vi "Six Lead ECG Monitor.vi"() -> ()   [LabVIEW 2013]
uses:
  SerialReadStateEnum.ctl
  <vilib>/Utility/file.llb/Write To Spreadsheet File (DBL).vi
  <vilib>/Instr/_visa.llb/VISA Configure Serial Port (Instr).vi
panel:
  out "unsigned byte array":u8[](array[numeric])
  out "size(s)":i32[](array[numeric])
  out "Saved File Path":path
  in  "File Name":string="ecgEarlobe2.txt"
  out "Sync 0":u8=165
  out "Sync 1":u8=90
  out "Protocol Version":u8=2
  out "End Packet":u8=1
  out "Parity":u16(ring) items=["None", "Odd", "Even", "Mark", "Space"]
  out "Stop Bits":u16(ring)=10 items=["1.0"=10, "1.5"=15, "2.0"=20]
  out "Flow Control":u16(ring) items=["None"=0, "XON/XOFF"=1, "RTS/CTS"=2, "DTR/DSR"=4]
  out "Current State":T1
  out "ECG/\nEMG":cluster{u16, u16, u16, u16, u16, u16}(graph)
  out "Count":u8
  out "Byte Count":u32=17
  in  "Stop":bool
  out "Data Bits":u16=8 min=5 max=8 step=1
  in  "VISA resource name":refnum<visa-resource-name>="COM3"
  out "Baud Rate":u32=57600
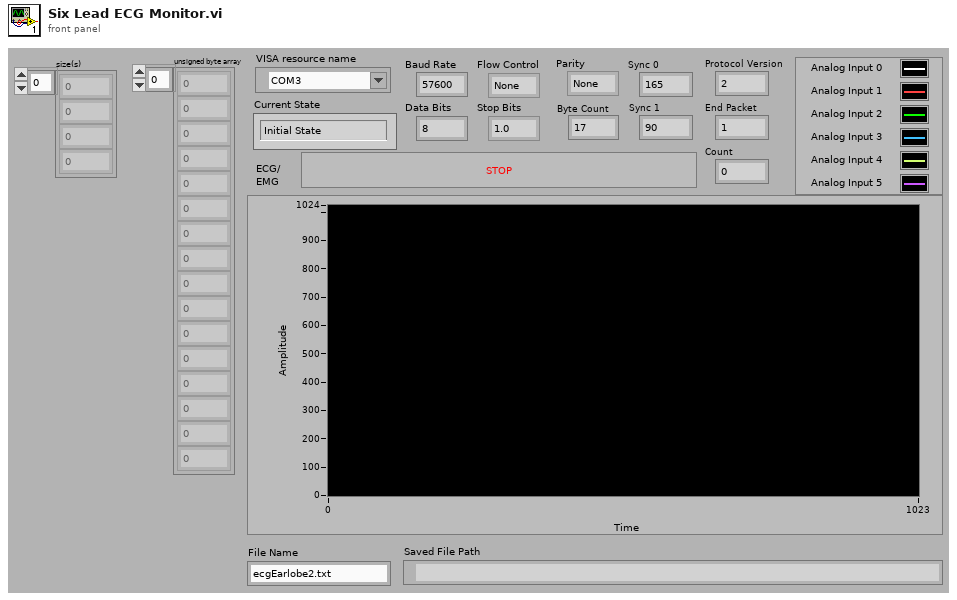
[diagram p1: front panel]
types:
  T1 = typedef "SerialReadStateEnum.ctl" = enum16{"Initial State", "Offset Corrected"}
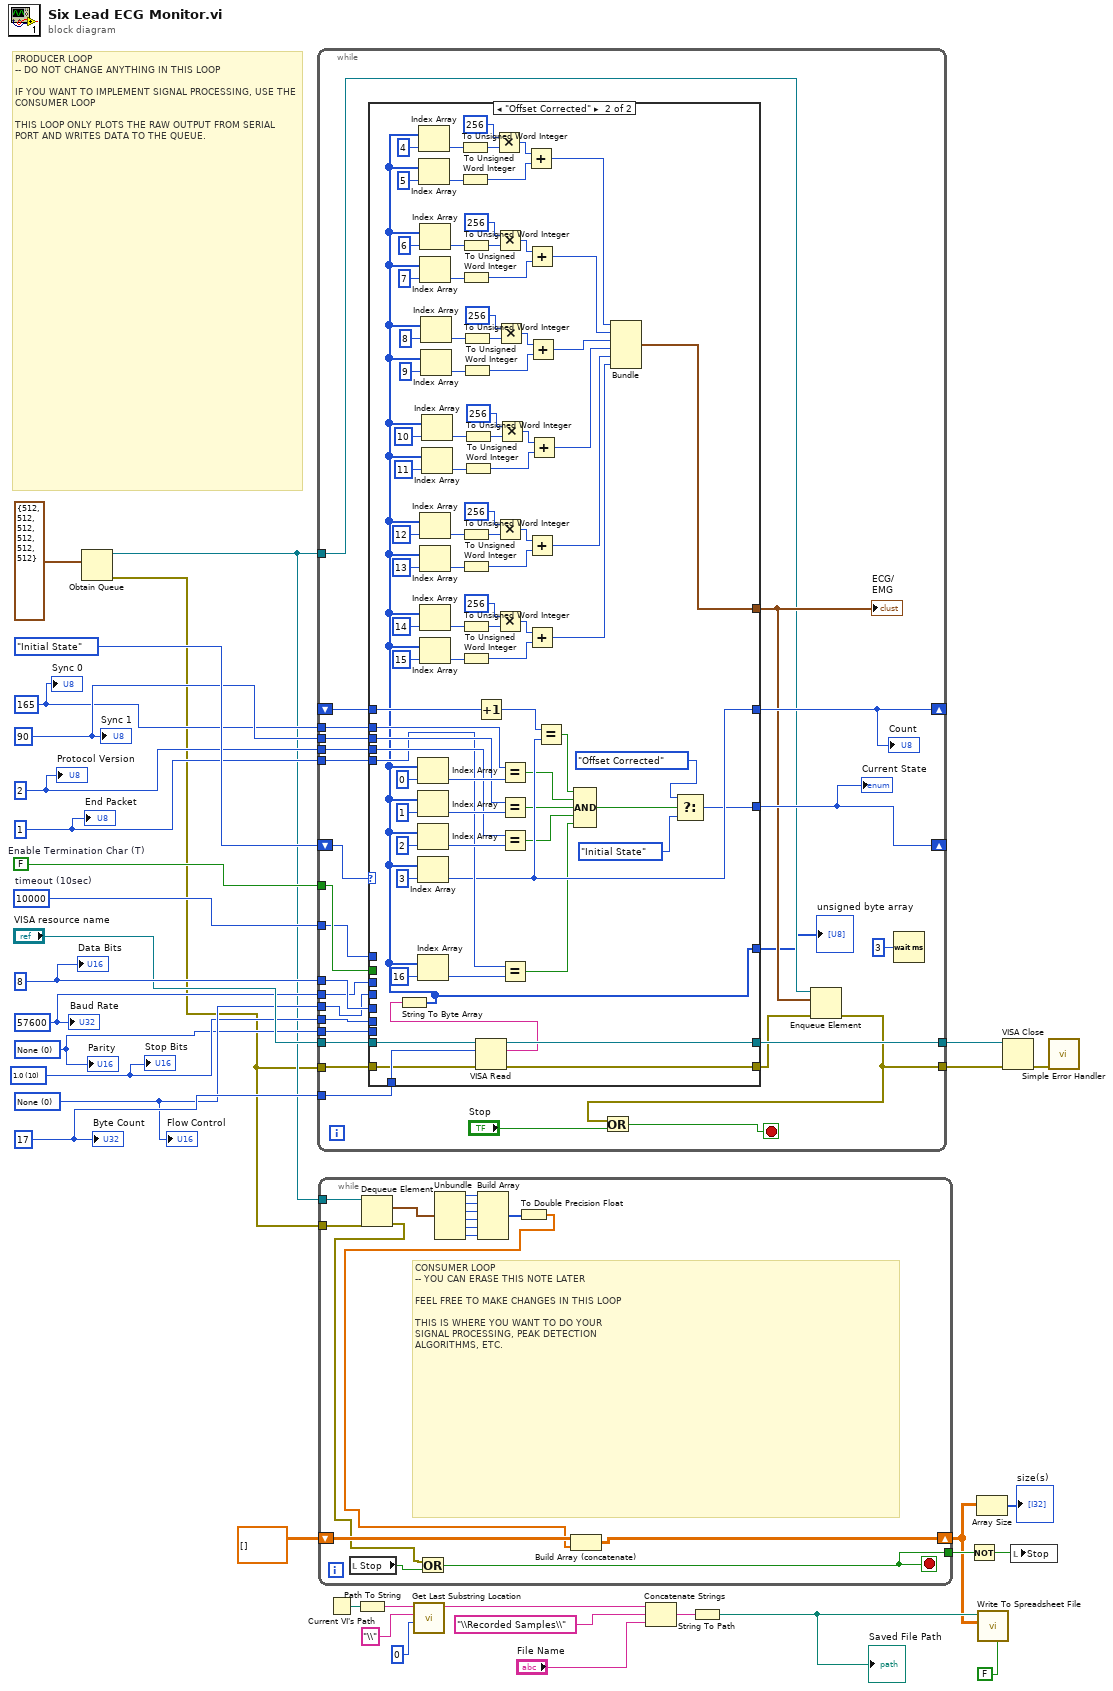
[diagram p0: block diagram]
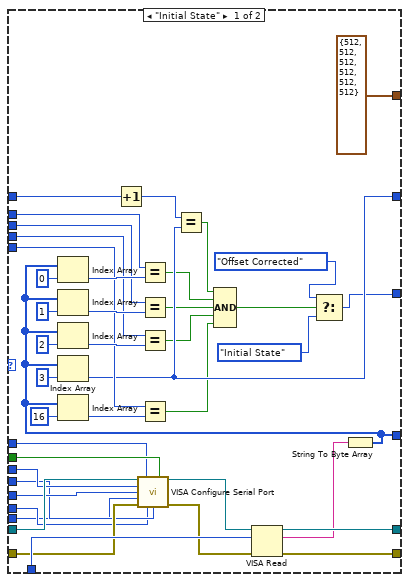
[diagram p2: hidden frame]
diagram:
  w27 = u8 165 ("Sync 0")
  w28 = u8 90 ("Sync 1")
  w29 = u8 2 ("Protocol Version")
  w30 = u8 1 ("End Packet")
  w23 = u16 8 ("Data Bits")
  w21 = u32 57600 ("Baud Rate")
  w18 = u16 0 items=["None", "Odd", "Even", "Mark", "Space"] ("Parity")
  w19 = u16 10 items=["1.0"=10, "1.5"=15, "2.0"=20] ("Stop Bits")
  w20 = u16 0 items=["None"=0, "XON/XOFF"=1, "RTS/CTS"=2, "DTR/DSR"=4] ("Flow Control")
  w31 = u32 17
  w25 = FALSE  # Enable Termination Char (T)
  w24 = u32 10000  # timeout (10sec)
  # "PRODUCER LOOP \n-- DO NOT CHANGE ANYTHING IN THIS LOOP\n\nIF YOU WANT TO IMPLEMENT SIGNAL PROCESSING, USE THE CONSUMER LOOP\n\nTHIS LOOP ONLY PLOTS THE RAW OUTPUT FROM SERIAL PORT AND WRITES DATA TO THE QUEUE."
  n1 = Obtain Queue(element data type=cluster{u16, u16, u16, u16, u16, u16} {512, 512, 512, 512, 512, 512}) -> (queue out=w17:refnum<queue>, error out=w6:errorcluster)  [unwired: 4 in, 1 out]
  n2 = while {
    tunnel: w6 -> [w60]
    tunnel: "VISA resource name" -> [w62]
    tunnel: w31 -> [w61]
    tunnel: [w59] -> w34
    tunnel: [w46] -> w35
    tunnel: w27 -> [w58]
    tunnel: w28 -> [w57]
    tunnel: w29 -> [w56]
    tunnel: w30 -> [w55]
    shift-right: [w53] -> _
    shift-left: _ -> [w54]
    shift-right: [w49] -> _
    shift-left: SerialReadStateEnum."Initial State" ("Enum") -> [w50]
    tunnel: w17 -> [w44]
    tunnel: w25 -> [w43]
    tunnel: w24 -> [w42]
    tunnel: w23 -> [w41]
    tunnel: w21 -> [w40]
    tunnel: w20 -> [w39]
    tunnel: w19 -> [w38]
    tunnel: w18 -> [w37]
    stop <- w52 stop-if-true
    n3 = case shown="\"Offset Corrected\"" w50 {
      tunnel: w62 -> [w73 w191]
      tunnel: w61 -> [w104 w190]
      tunnel: w60 -> [w74 w189]
      tunnel: [w103 w188] -> w59
      tunnel: w58 -> [w92 w177]
      tunnel: w57 -> [w91 w176]
      tunnel: w56 -> [w90 w175]
      tunnel: w55 -> [w89 w174]
      tunnel: w54 -> [w88 w173]
      tunnel: [w86 w171] -> w53
      tunnel: [w80 w165] -> w47
      tunnel: [w76 w161] -> w49
      tunnel: [cluster{u16, u16, u16, u16, u16, u16} {512, 512, 512, 512, 512, 512} w106] -> w45
      tunnel: w43 -> [w70 _]
      tunnel: w42 -> [w69 _]
      tunnel: w41 -> [w68 _]
      tunnel: w40 -> [w67 _]
      tunnel: w39 -> [w66 _]
      tunnel: w38 -> [w65 _]
      tunnel: w37 -> [w64 _]
      tunnel: [w63 w105] -> w36
      frame "Initial State" {
        n4 = Increment(x=w88) -> (x+1=w87:u8)
        n5 = call-poly "VISA Configure Serial Port"("VISA resource name"=w73, "timeout (10sec)"=w69, "Enable Termination\nChar (T)"=w70, "baud rate (9600)"=w67, "data bits (8)"=w68, "parity (0:none)"=w64, "error in (no error)"=w74, "stop bits (10: 1 bit)"=w65, "flow control (0:none)"=w66) -> ("VISA resource name out"=w71:refnum<visa-resource-name>, "error out"=w72:errorcluster)  [unwired: 5 out]
        n6 = VISA Read(VISA resource name=w71, byte count=w104, error in (no error)=w72) -> (VISA resource name out=w103:refnum<visa-resource-name>, read buffer=w102:string, error out=w80:errorcluster)  [unwired: 1 out]
        n7 = String To Byte Array(string=w102) -> (unsigned byte array=w63:u8[])
        n8 = Index Array(array=w63, index=0) -> (element=w96:u8)
        n9 = Index Array(array=w63, index=1) -> (element=w95:u8)
        n10 = Index Array(array=w63, index=2) -> (element=w94:u8)
        n11 = Index Array(array=w63, index=3) -> (element=w86:u8)
        n12 = Index Array(array=w63, index=16) -> (element=w93:u8)
        n13 = Equal?(x=w92, y=w96) -> (x = y?=w84:bool)
        n14 = Equal?(x=w91, y=w95) -> (x = y?=w83:bool)
        n15 = Equal?(x=w90, y=w94) -> (x = y?=w82:bool)
        n16 = Equal?(x=w89, y=w93) -> (x = y?=w81:bool)
        n17 = Equal?(x=w87, y=w86) -> (x = y?=w85:bool)
        n18 = Compound Arithmetic op=AND(w85, w84, w83, w82, w81) -> (w77:bool)
        n19 = Select(t=SerialReadStateEnum."Offset Corrected" ("Enum"), s=w77, f=SerialReadStateEnum."Initial State" ("Enum")) -> (s? t:f=w76:T1)
      }
      frame "Offset Corrected" {
        n20 = Increment(x=w173) -> (x+1=w172:u8)
        n21 = VISA Read(VISA resource name=w191, byte count=w190, error in (no error)=w189) -> (VISA resource name out=w188:refnum<visa-resource-name>, read buffer=w187:string, error out=w165:errorcluster)  [unwired: 1 out]
        n22 = String To Byte Array(string=w187) -> (unsigned byte array=w105:u8[])
        n23 = Index Array(array=w105, index=0) -> (element=w181:u8)
        n24 = Index Array(array=w105, index=1) -> (element=w180:u8)
        n25 = Index Array(array=w105, index=2) -> (element=w179:u8)
        n26 = Index Array(array=w105, index=3) -> (element=w171:u8)
        n27 = Index Array(array=w105, index=16) -> (element=w178:u8)
        n28 = Index Array(array=w105, index=4) -> (element=w117:u8)
        n29 = Index Array(array=w105, index=5) -> (element=w115:u8)
        n30 = Index Array(array=w105, index=6) -> (element=w124:u8)
        n31 = Index Array(array=w105, index=7) -> (element=w126:u8)
        n32 = Index Array(array=w105, index=12) -> (element=w149:u8)
        n33 = Index Array(array=w105, index=13) -> (element=w147:u8)
        n34 = Index Array(array=w105, index=14) -> (element=w156:u8)
        n35 = Index Array(array=w105, index=15) -> (element=w158:u8)
        n36 = Index Array(array=w105, index=8) -> (element=w133:u8)
        n37 = Index Array(array=w105, index=9) -> (element=w131:u8)
        n38 = Index Array(array=w105, index=10) -> (element=w140:u8)
        n39 = Index Array(array=w105, index=11) -> (element=w142:u8)
        n40 = To Unsigned Word Integer(number=w117) -> (unsigned 16bit integer=w116:u16)
        n41 = To Unsigned Word Integer(number=w115) -> (unsigned 16bit integer=w114:u16)
        n42 = To Unsigned Word Integer(number=w124) -> (unsigned 16bit integer=w125:u16)
        n43 = To Unsigned Word Integer(number=w126) -> (unsigned 16bit integer=w127:u16)
        n44 = To Unsigned Word Integer(number=w149) -> (unsigned 16bit integer=w148:u16)
        n45 = To Unsigned Word Integer(number=w147) -> (unsigned 16bit integer=w146:u16)
        n46 = To Unsigned Word Integer(number=w156) -> (unsigned 16bit integer=w157:u16)
        n47 = To Unsigned Word Integer(number=w158) -> (unsigned 16bit integer=w159:u16)
        n48 = To Unsigned Word Integer(number=w133) -> (unsigned 16bit integer=w132:u16)
        n49 = To Unsigned Word Integer(number=w131) -> (unsigned 16bit integer=w130:u16)
        n50 = To Unsigned Word Integer(number=w140) -> (unsigned 16bit integer=w141:u16)
        n51 = To Unsigned Word Integer(number=w142) -> (unsigned 16bit integer=w143:u16)
        n52 = Multiply(x=u16 256, y=w116) -> (x*y=w113:u16)
        n53 = Multiply(x=u16 256, y=w125) -> (x*y=w128:u16)
        n54 = Multiply(x=u16 256, y=w148) -> (x*y=w145:u16)
        n55 = Multiply(x=u16 256, y=w157) -> (x*y=w160:u16)
        n56 = Multiply(x=u16 256, y=w132) -> (x*y=w129:u16)
        n57 = Multiply(x=u16 256, y=w141) -> (x*y=w144:u16)
        n58 = Equal?(x=w177, y=w181) -> (x = y?=w169:bool)
        n59 = Equal?(x=w176, y=w180) -> (x = y?=w168:bool)
        n60 = Equal?(x=w175, y=w179) -> (x = y?=w167:bool)
        n61 = Equal?(x=w174, y=w178) -> (x = y?=w166:bool)
        n62 = Add(x=w113, y=w114) -> (x+y=w107:u16)
        n63 = Add(x=w128, y=w127) -> (x+y=w108:u16)
        n64 = Add(x=w145, y=w146) -> (x+y=w111:u16)
        n65 = Add(x=w160, y=w159) -> (x+y=w112:u16)
        n66 = Add(x=w129, y=w130) -> (x+y=w109:u16)
        n67 = Add(x=w144, y=w143) -> (x+y=w110:u16)
        n68 = Equal?(x=w172, y=w171) -> (x = y?=w170:bool)
        n69 = Compound Arithmetic op=AND(w170, w169, w168, w167, w166) -> (w164:bool)
        n70 = Bundle(w107, w108, w109, w110, w111, w112) -> (w106:cluster{u16, u16, u16, u16, u16, u16})  [unwired: 1 in]
        n71 = Select(t=SerialReadStateEnum."Offset Corrected" ("Enum"), s=w164, f=SerialReadStateEnum."Initial State" ("Enum")) -> (s? t:f=w161:T1)
      }
    }
    "Count" <- w53
    "ECG/\nEMG" <- w45
    "Current State" <- w49
    "unsigned byte array" <- w36
    n72 = Enqueue Element(queue=w44, element=w45, error in (no error)=w47) -> (error out=w46:errorcluster)  [unwired: 1 in, 2 out]
    n73 = Or(x=w46, y="Stop") -> (x .or. y?=w52:bool)
    n74 = Wait (ms)(milliseconds to wait=u32 3) -> ()  [unwired: 1 out]
  }
  n75 = while {
    tunnel: w17 -> [w207]
    tunnel: w6 -> [w206]
    shift-right: [w195] -> w2
    shift-left: dbl[][] [] -> [w197]
    tunnel: [w194] -> w4
    stop <- w194 stop-if-true
    # "CONSUMER LOOP\n-- YOU CAN ERASE THIS NOTE LATER\n\nFEEL FREE TO MAKE CHANGES IN THIS LOOP\n\nTHIS IS WHERE YOU WANT TO DO YOUR \nSIGNAL PROCESSING, PEAK DETECTION \nALGORITHMS, ETC."
    n76 = local read "Stop"() -> (w205:bool)
    n77 = Dequeue Element(queue=w207, error in (no error)=w206) -> (element=w204:cluster{u16, u16, u16, u16, u16, u16}, error out=w193:errorcluster)  [unwired: 1 in, 2 out]
    n78 = Or(x=w193, y=w205) -> (x .or. y?=w194:bool)
    n79 = Unbundle(w204) -> (w203:u16, w202:u16, w201:u16, w200:u16, w199:u16, w198:u16)
    n80 = Build Array(w203, w202, w201, w200, w199, w198) -> (w196:u16[])
    n81 = To Double Precision Float(number=w196) -> (double precision float=w192:dbl[])
    n82 = Build Array (concatenate)(w197, w192) -> (w195:dbl[][])
  }
  n83 = Current VI's Path() -> (path=w16:path)
  n84 = Path To String(path=w16) -> (string=w15:string)
  n85 = call "Get Last Substring Location.vi"("offset (0)"=0, "regular expression"="\\", "string"=w15) -> ("before substring"=w12:string)  [unwired: 5 in, 3 out]
  n86 = Concatenate Strings(w12, "\\Recorded Samples\\" ("string"), "File Name") -> (w10:string)
  n87 = String To Path(string=w10) -> (path=w7:path)
  "Saved File Path" <- w7
  n88 = Not(x=w4) -> (.not. x?=w3:bool)
  n89 = Array Size(array=w2) -> (size(s)=→"size(s)":i32[])
  n90 = call-poly <vilib>:"Write To Spreadsheet File.vi"("transpose? (no:F)"=FALSE, "2D data"=w2, "file path (dialog if empty)"=w7) -> ()  [unwired: 5 in, 1 out]
  n91 = VISA Close(VISA resource name=w34, error in (no error)=w35) -> (error out=w33:errorcluster)
  n92 = local write "Stop"(w3) -> ()
  n93 = call <vilib>:"Simple Error Handler.vi"("error in (no error)"=w33) -> ()  [unwired: 1 in, 8 out]
  "Baud Rate" <- w21
  "Data Bits" <- w23
  "Byte Count" <- w31
  "Flow Control" <- w20
  "Stop Bits" <- w19
  "Parity" <- w18
  "End Packet" <- w30
  "Protocol Version" <- w29
  "Sync 1" <- w28
  "Sync 0" <- w27
